vi "OAT Edge Detection (N Tach).vi"(5 "reset? (True)":bool=TRUE, 6 "sampling frequency [Hz]":dbl[](array[numeric]), 7 "missing pulses? (no:F)":bool[](array[boolean]), 8 "slope (Rising)":u16[](array[ring]) items=["Rising", "Falling"], 9 "pulse width (2)":i32[](array[numeric]), 10 "threshold (0.0)":dbl[](array[numeric]) format="%.2f", 11 "x(n)":cluster{"Y":dbl[]}[](array[cluster]) {"Y" format="%.2f"}) -> (0 "number of pulses":i32[](array[numeric]), 3 "pulse position [s]":cluster{dbl[]}[](array[cluster]) {"?" format="%.2f"})   [LabVIEW 2017, in "SoundVib_TachProcess.lvlib"]
doc: "Detects the edges in the tachometer pulses contained in <B>x[n]</B> that cross <B>threshold</B>. Perform edge detection to determine the tachometer pulse position. The VI recognizes the points where the signal crosses <B>threshold</B> and <B>x[n]</B> as edges. The VI returns the locations of the detected edges in <B>pulse positions [s]</B>."
uses:
  <vilib>/addons/Sound and Vibration/Order Analysis/Tach Process/SoundVib_TachProcess.lvlib
  <vilib>/Analysis/8numeric.llb/Threshold Detector.vi
panel:
  # "Edge Detection (N Tach)"
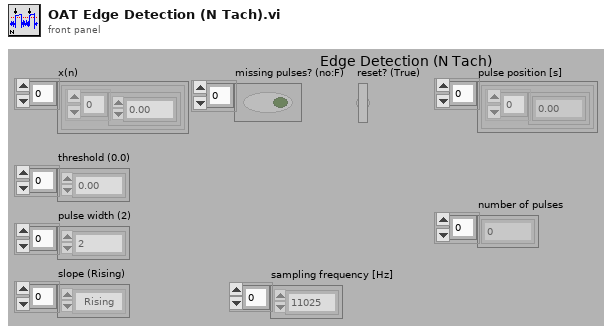
[diagram p1: front panel]
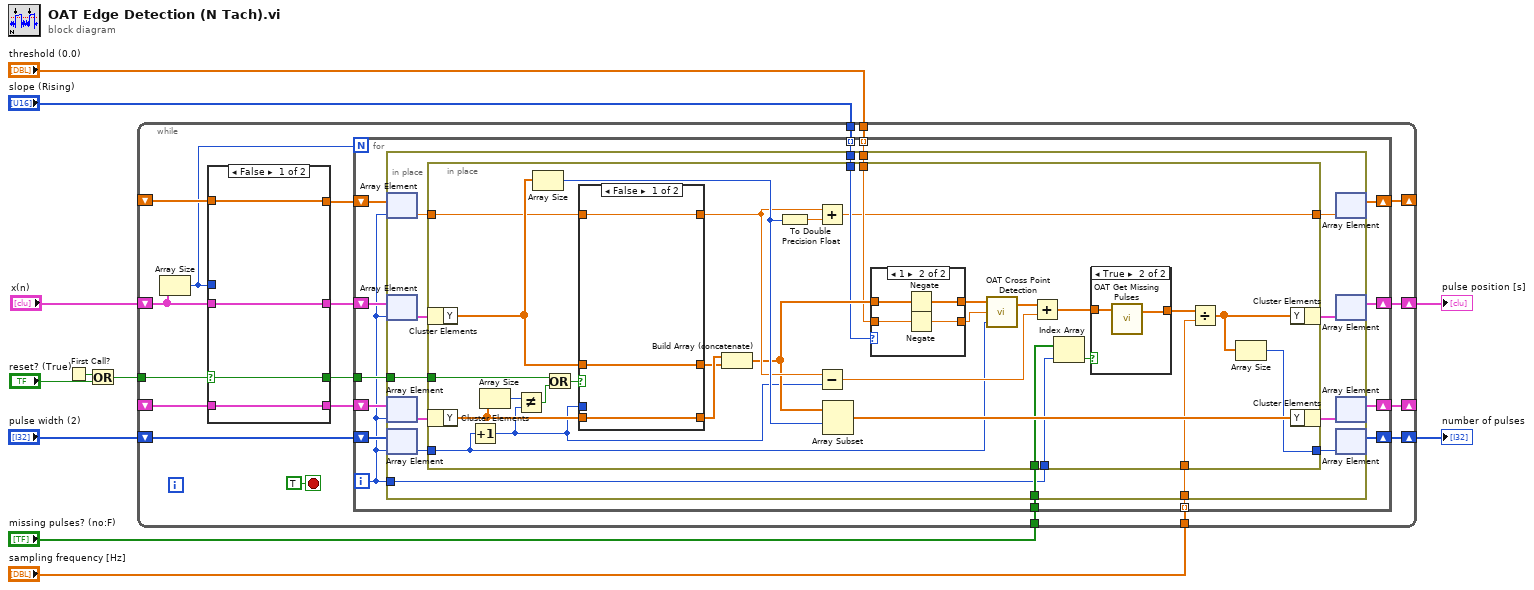
[diagram p0: block diagram]
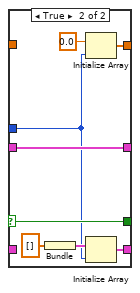
[diagram p2: hidden frame]
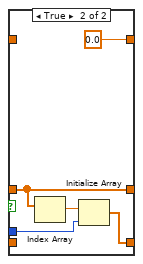
[diagram p5: hidden frame]
diagram:
  n1 = First Call?() -> (First Call?: T/F=w10:bool)
  n2 = Or(x=w10, y="reset? (True)") -> (x .or. y?=w11:bool)
  n3 = while {
    shift-right: [w29] -> _
    shift-left: _ -> [w25]
    tunnel: w11 -> [w26]
    shift-right: [w27] -> _
    shift-left: _ -> [w24]
    tunnel: "threshold (0.0)" -> [w17]
    tunnel: "slope (Rising)" -> [w16]
    tunnel: "missing pulses? (no:F)" -> [w15]
    tunnel: "sampling frequency [Hz]" -> [w14]
    shift-right: [w28] -> w3
    shift-left: "x(n)" -> [w19]
    shift-right: [w13] -> w2
    shift-left: "pulse width (2)" -> [w12]
    stop <- TRUE stop-if-true
    n4 = Array Size(array=w19) -> (size(s)=w18:i32)
    n5 = case shown="False" w26 {
      selector: w26 -> [w31 w36]
      tunnel: w25 -> [w32 _]
      tunnel: w24 -> [w33 _]
      tunnel: w19 -> [w34 w42]
      tunnel: [w34 w42] -> w23
      tunnel: [w33 w40] -> w22
      tunnel: [w32 w37] -> w21
      tunnel: [w31 w36] -> w20
      tunnel: w18 -> [_ w35]
      frame False {
      }
      frame True {
        n6 = Bundle("Y"=dbl[] []) -> (w38:cluster{"Y":dbl[]})  [unwired: 1 in]
        n7 = Initialize Array(0.0 ("element"), w35) -> (w40:dbl[])
        n8 = Initialize Array(w38, w35) -> (w37:cluster{"Y":dbl[]}[])
      }
    }
    n9 = for {
      N: w18 -> [_]
      tunnel: w20 -> [w56]
      shift-right: [w54] -> w27
      shift-left: w22 -> [w55]
      shift-right: [w52] -> w28
      shift-left: w23 -> [w53]
      shift-right: [w50] -> w29
      shift-left: w21 -> [w51]
      tunnel: w17 -> [w49] mode=indexing
      tunnel: w16 -> [w48] mode=indexing
      tunnel: w15 -> [w47]
      tunnel: w14 -> [w46] mode=indexing
      shift-right: [w43] -> w13
      shift-left: w12 -> [w45]
      i -> [w44]
      n10 = in-place {
        in-place-border: w56 -> [w70]
        in-place-border: w44 -> [w60]
        in-place-border: w49 -> [w63]
        in-place-border: w48 -> [w62]
        in-place-border: w47 -> [w61]
        in-place-border: w46 -> [w59]
        n11 = in-place-array #1(w55, w44) -> (w65:dbl)
        n12 = in-place-array #2(w53, w44) -> (w69:cluster{"Y":dbl[]})
        n13 = in-place-array #3(w51, w44) -> (w68:cluster{"Y":dbl[]})
        n14 = in-place-array #4(w45, w44) -> (w58:i32)
        n15 = in-place {
          in-place-border: w70 -> [w99]
          in-place-border: w65 -> [w90]
          in-place-border: [w73] -> w64
          in-place-border: w63 -> [w80]
          in-place-border: w62 -> [w79]
          in-place-border: w61 -> [w76]
          in-place-border: w60 -> [w77]
          in-place-border: w59 -> [w75]
          in-place-border: [w74] -> w57
          in-place-border: w58 -> [w72]
          n16 = in-place-cluster #5(w69) -> ("Y"=w96:dbl[])
          n17 = in-place-cluster #6(w68) -> ("Y"=w94:dbl[])
          n18 = Increment(x=w72) -> (x+1=w71:i32)
          n19 = Array Size(array=w94) -> (size(s)=w101:i32)
          n20 = Not Equal?(x=w101, y=w71) -> (x != y?=w100:bool)
          n21 = Array Size(array=w96) -> (size(s)=w91:i32)
          n22 = Or(x=w99, y=w100) -> (x .or. y?=w93:bool)
          n23 = case shown="False" w93 {
            tunnel: [w112 w116] -> w98
            tunnel: w96 -> [w113 w115]
            tunnel: w71 -> [_ w117]
            tunnel: [w113 w115] -> w97
            tunnel: w94 -> [w112 _]
            tunnel: [w111 0.0 ("t")] -> w89
            tunnel: w90 -> [w111 _]
            frame False {
            }
            frame True {
              n24 = Index Array(array=w115) -> (element=w118:dbl)  [unwired: 1 in]
              n25 = Initialize Array(w118, w117) -> (w116:dbl[])
            }
          }
          n26 = Build Array (concatenate)(w98, w97) -> (w82:dbl[])
          n27 = To Double Precision Float(number=w91) -> (double precision float=w92:dbl)
          n28 = Add(x=w89, y=w92) -> (x+y=w73:dbl)
          n29 = Subtract(x=w89, y=w71) -> (x-y=w78:dbl)
          n30 = Array Subset(array=w82, index=w91) -> (w95:dbl[])  [unwired: 1 in]
          n31 = case shown="1" w79 {
            tunnel: w80 -> [w105 w108]
            tunnel: w82 -> [w106 w110]
            tunnel: [w106 w109] -> w87
            tunnel: [w105 w107] -> w88
            frame 0, Default {
            }
            frame 1 {
              n32 = Negate(x=w110) -> (-x=w109:dbl[])
              n33 = Negate(x=w108) -> (-x=w107:dbl)
            }
          }
          n34 = call <vilib>:"OAT Cross Point Detection.vi"("pulse width (2)"=w72, "threshold (0)"=w88, "data in"=w87) -> ("edge position"=w86:dbl[])  [unwired: 1 in]
          n35 = Add(x=w86, y=w78) -> (x+y=w84:dbl[])
          n36 = Index Array(array=w76, index=w77) -> (element=w83:bool)
          n37 = case shown="True" w83 {
            tunnel: w84 -> [w102 w103]
            tunnel: [w102 w104] -> w85
            frame False {
            }
            frame True {
              n38 = call <vilib>:"OAT Get Missing Pulses.vi"("pulse positions"=w103) -> ("modified pulse positions"=w104:dbl[])  [unwired: 1 in, 1 out]
            }
          }
          n39 = Divide(x=w85, y=w75) -> (x/y=w81:dbl[])
          n40 = Array Size(array=w81) -> (size(s)=w74:i32)
          n41 = in-place-cluster #5("Y"=w81) -> (w66:cluster{"Y":dbl[]})
          n42 = in-place-cluster #6("Y"=w95) -> (w67:cluster{"Y":dbl[]})
        }
        n43 = in-place-array #1(w64) -> (w54:dbl[])  [unwired: 1 out]
        n44 = in-place-array #2(w66) -> (w52:cluster{"Y":dbl[]}[])  [unwired: 1 out]
        n45 = in-place-array #3(w67) -> (w50:cluster{"Y":dbl[]}[])  [unwired: 1 out]
        n46 = in-place-array #4(w57) -> (w43:i32[])  [unwired: 1 out]
      }
    }
  }
  "number of pulses" <- w2
  "pulse position [s]" <- w3
